vi "실습2-8 문자열 함수.vi"() -> ()   [LabVIEW 2014]
panel:
  out "이전 부분 문자열":string
  out "숫자":dbl
  out "부분 문자열":string
  out "길이":i32
  out "문자열 2":string
  in  "문자열":string
  # "*문자열 연결"
  # "*문자열 잘라내기\nex) PLC 통신"
  # "*패턴일치\nex) GPIB 통신"
  # "hello world!"
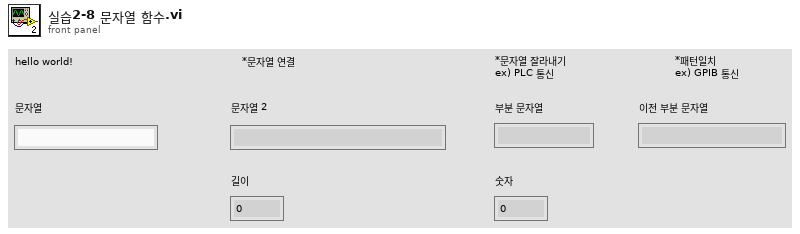
[diagram p1: front panel]
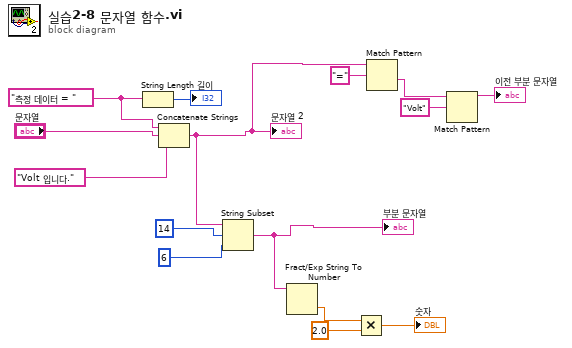
[diagram p0: block diagram]
diagram:
  w13 = "측정 데이터 = " ("문자열")
  n1 = String Length(string=w13) -> (length=→"길이":i32)
  n2 = Concatenate Strings(w13, "문자열", "Volt 입니다." ("문자열")) -> (w1:string)
  "문자열 2" <- w1
  n3 = String Subset(string=w1, offset (0)=14 ("오프셋(0)"), length (rest)=6 ("길이(나머지)")) -> (substring=w6:string)
  "부분 문자열" <- w6
  n4 = Fract/Exp String To Number(string=w6) -> (number=w9:dbl)  [unwired: 3 in, 1 out]
  n5 = Multiply(x=w9, y=2.0) -> (x*y=→"숫자":dbl)
  n6 = Match Pattern(string=w1, regular expression="=" ("정규식")) -> (after substring=w4:string)  [unwired: 1 in, 3 out]
  n7 = Match Pattern(string=w4, regular expression="Volt" ("정규식")) -> (before substring=→"이전 부분 문자열":string)  [unwired: 1 in, 3 out]
